vi "XYZStage Message Loop.vi"(8 "error in (no error)":errorcluster, 9 "Data Queue":refnum<queue>, 10 "Stage Readout Notifier":refnum<notifier>, 11 "Message Queues":T1) -> (0 "error out":errorcluster)   [LabVIEW 2015, in "XYZStage.lvlib"]
uses:
  XYZStage.lvlib
  support/Message Queue/All Message Queues.ctl
  support/Message Queue/Message Cluster.ctl
  XYZStage Configuration.ctl
  XYZStage State.ctl
  XYZStage Loop State.ctl
  <vilib>/Utility/error.llb/Error Cluster From Error Code.vi
  <vilib>/ErrorRing/Error Ring.xnode
  support/Message Queue/Message Queue.lvlib
panel:
  out "XYZ Microns":dbl[](array[numeric])
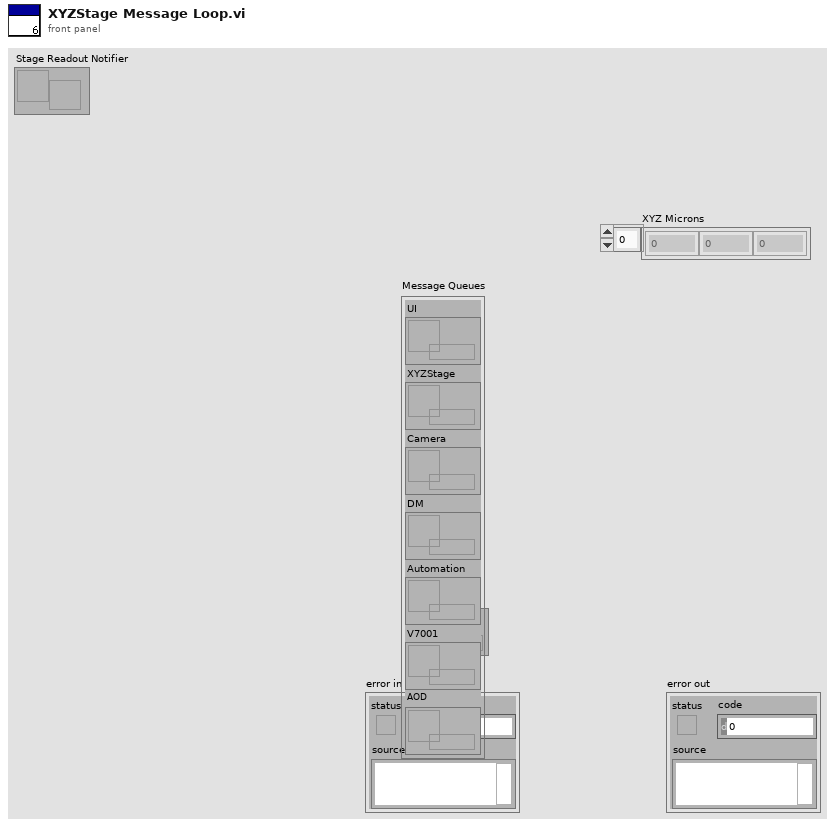
[diagram p1: front panel]
types:
  T1 = typedef "Message Queue.lvlib/All Message Queues.ctl" = cluster{"UI":refnum<queue>, "XYZStage":refnum<queue>, "Camera":refnum<queue>, "DM":refnum<queue>, "Automation":refnum<queue>, "V7001":refnum<queue>, "AOD":refnum<queue>}
  T2 = typedef "XYZStage.lvlib/XYZStage State.ctl" = cluster{"XYZStage State":T3, "Handle out":u32, "VISA resource name":refnum<visa-resource-name>, "num controllers connected":u8, "Connector statuses":u8[], "Position in Microns":dbl[], "measured manipulator":u8}
  T3 = typedef "XYZStage.lvlib/XYZStage Loop State.ctl" = enum16{"Idle", "Connected", "Moving"}
  T4 = typedef "XYZStage.lvlib/XYZStage Configuration.ctl" = cluster{"VISA resource name":refnum<visa-resource-name>, "Timeout (3sec)":u32}
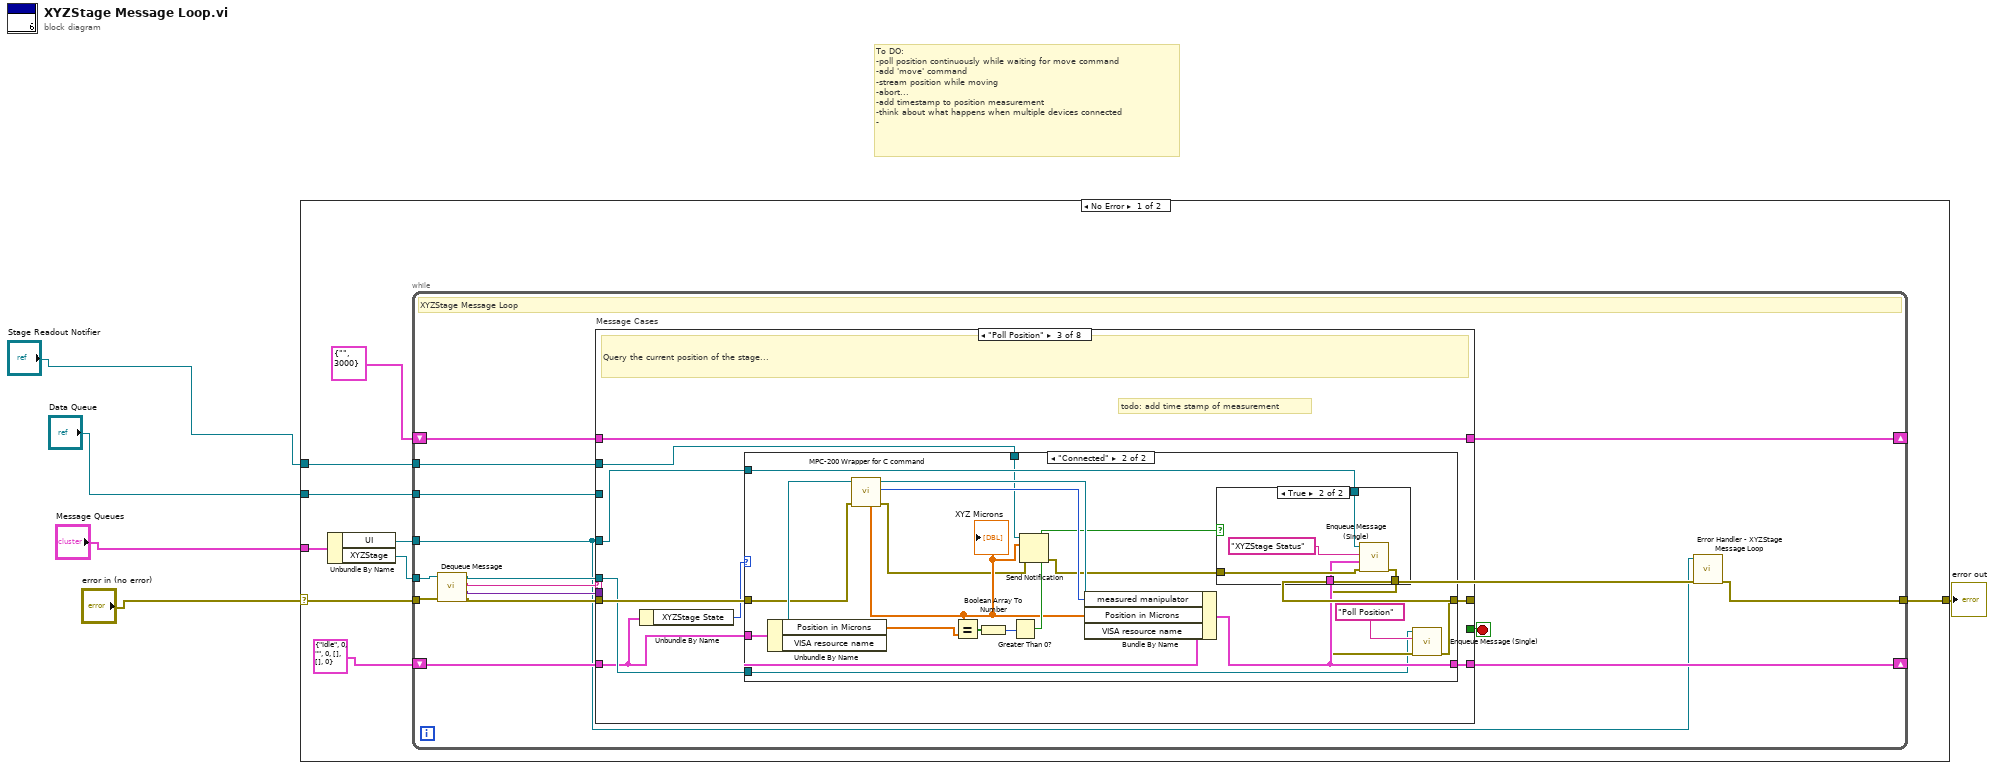
[diagram p0: block diagram]
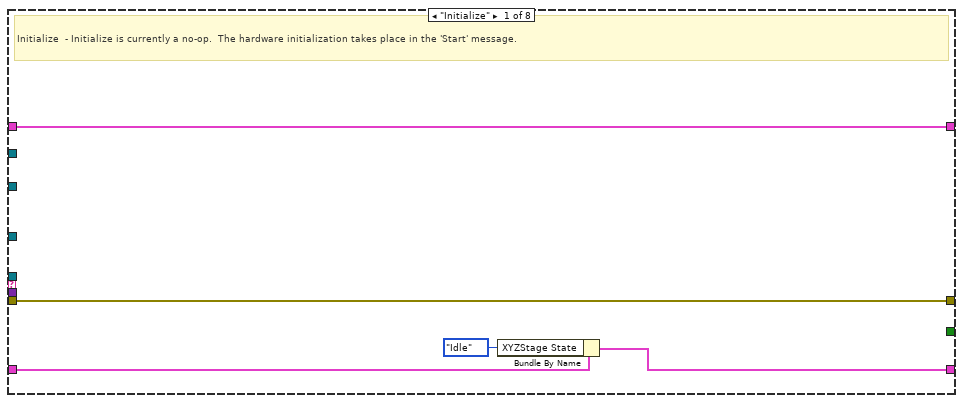
[diagram p2: hidden frame]
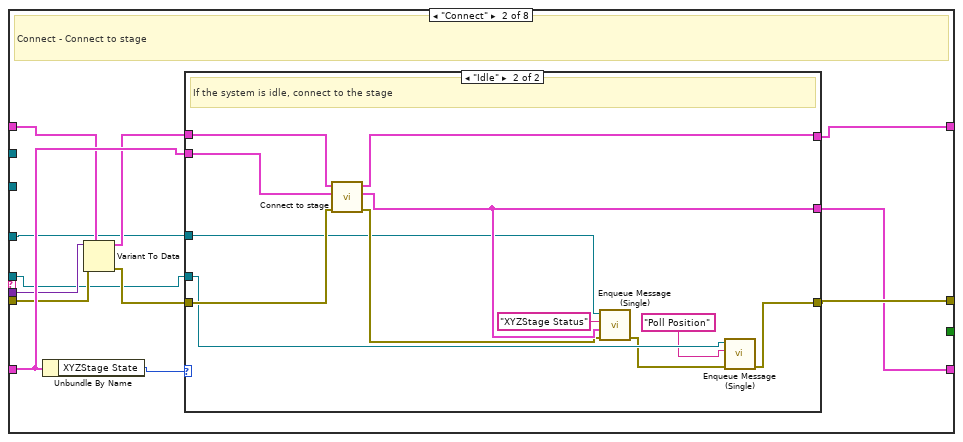
[diagram p3: hidden frame]
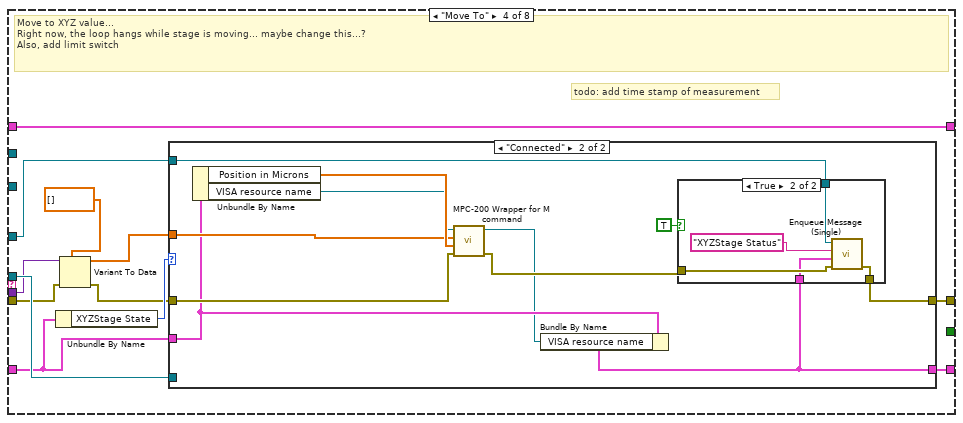
[diagram p7: hidden frame]
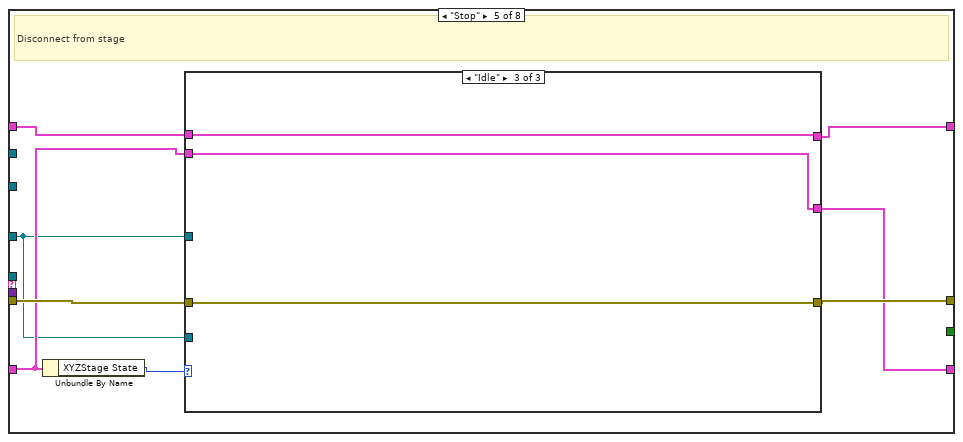
[diagram p10: hidden frame]
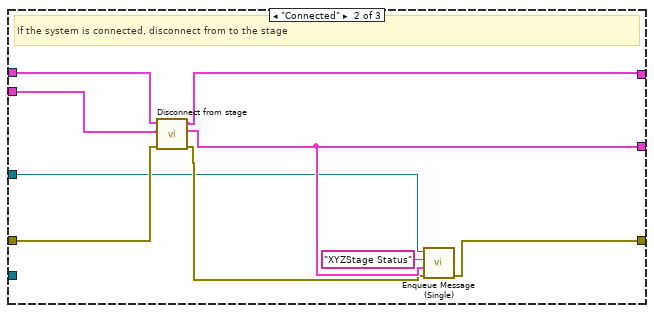
[diagram p12: hidden frame]
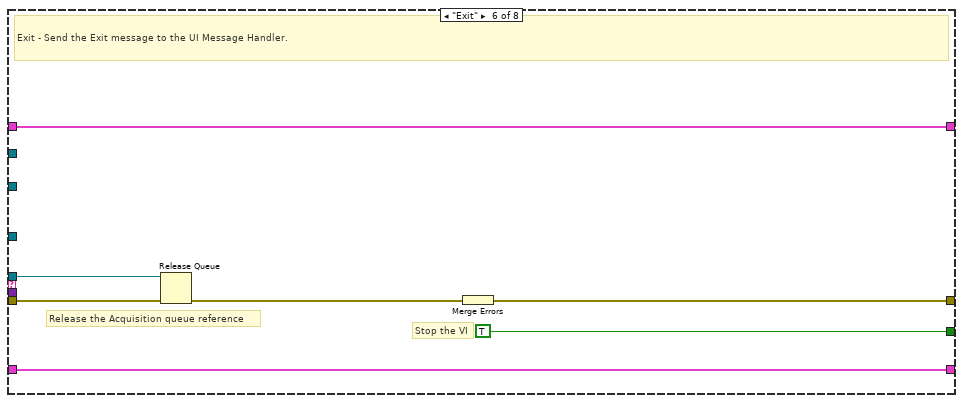
[diagram p13: hidden frame]
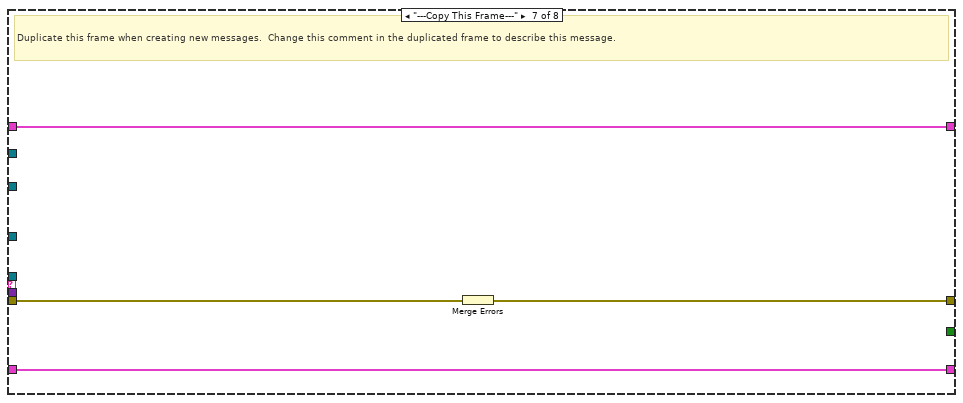
[diagram p14: hidden frame]
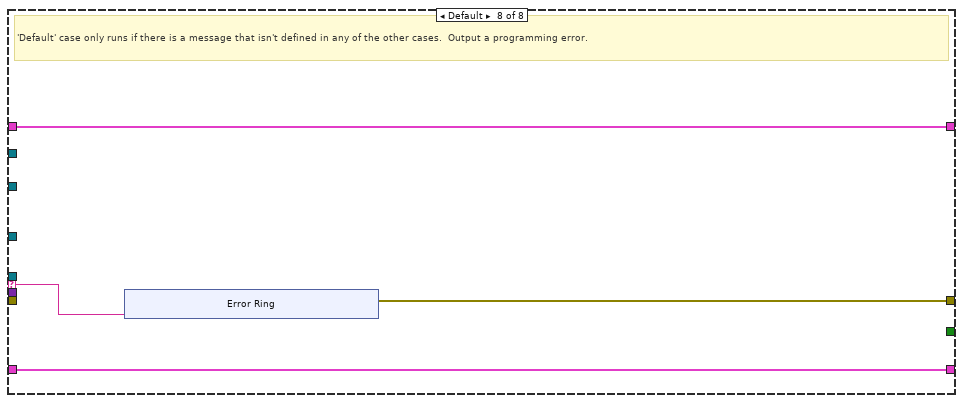
[diagram p15: hidden frame]
diagram:
  # "To DO:\n-poll position continuously while waiting for move command\n-add 'move' command\n-stream position while moving\n-abort...\n-add timestamp to position measurement\n-think about what happens when multiple devices connected\n-"
  n1 = case shown="No Error" "error in (no error)" {
    selector: "error in (no error)" -> [w11 w175]
    tunnel: "Message Queues" -> [w14 _]
    tunnel: [w12 w175] -> w5
    tunnel: "Stage Readout Notifier" -> [w9 _]
    tunnel: "Data Queue" -> [w8 _]
    frame No Error {
      n2 = Unbundle By Name(w14) -> ("UI"=w10:refnum<queue>, "XYZStage"=w13:refnum<queue>)
      n3 = while {
        tunnel: w13 -> [w23]
        shift-right: [w29] -> _
        shift-left: T4 {"VISA resource name"="", "Timeout (3sec)"=3000} ("Hardware Configuration") -> [w30]
        tunnel: w10 -> [w15]
        tunnel: w9 -> [w27]
        tunnel: w8 -> [w26]
        shift-right: [w24] -> _
        shift-left: T2 {"XYZStage State"=enum."Idle", "Handle out"=0, "VISA resource name"="", "num controllers connected"=0, "Connector statuses"=[], "Position in Microns"=[], "measured manipulator"=0} ("Cluster") -> [w25]
        tunnel: w11 -> [w22]
        tunnel: [w17] -> w12
        stop <- w28 stop-if-true
        # "XYZStage Message Loop"
        n4 = call "Dequeue Message.vi"("error in (no error)"=w22, "Message Queue"=w23) -> ("error out"=w18:errorcluster, "Message Data"=w19:variant, "Message"=w20:string, "dup Message Queue"=w21:refnum<queue>)  [unwired: 6 in]
        n5 = case "Message Cases" shown="\"Poll Position\"" w20 {
          selector: w20 -> [_ _ _ _ _ _ _ w164]
          tunnel: w21 -> [_ w36 w66 w106 _ w154 _ _]
          tunnel: w18 -> [w35 w38 w70 w103 w135 w156 w163 _]
          tunnel: [w35 w47 w67 w107 w137 w158 w161 w165] -> w16
          tunnel: w30 -> [w34 w42 w71 w110 w136 w157 w162 w167]
          tunnel: [w34 w45 w71 w110 w133 w157 w162 w167] -> w29
          tunnel: [_ _ _ _ _ TRUE _ _] -> w28
          tunnel: w19 -> [_ w40 _ w101 _ _ _ _]
          tunnel: w15 -> [_ w37 w69 w109 w130 _ _ _]
          tunnel: w27 -> [_ _ w63 _ _ _ _ _]
          tunnel: w26 -> [_ _ _ _ _ _ _ _]
          tunnel: w25 -> [w33 w43 w65 w105 w131 w153 w160 w166]
          tunnel: [w32 w46 w68 w108 w134 w153 w160 w166] -> w24
          frame "Initialize" {
            # "Initialize  - Initialize is currently a no-op.  The hardware initialization takes place in the 'Start' message."
            n6 = Bundle By Name(cluster=w33, "XYZStage State"=XYZStage_Loop_State."Idle") -> (w32:T2)
          }
          frame "Connect" {
            # "Connect - Connect to stage"
            n7 = Unbundle By Name(w43) -> ("XYZStage State"=w44:T3)
            n8 = Variant To Data(error in=w38, type=w42, Variant=w40) -> (data=w41:T4, error out=w39:errorcluster)
            n9 = case shown="\"Idle\"" w44 {
              tunnel: [w49 w51] -> w47
              tunnel: w41 -> [w50 w62]
              tunnel: w39 -> [w49 w60]
              tunnel: [w50 w61] -> w45
              tunnel: [w48 w57] -> w46
              tunnel: w43 -> [w48 w59]
              tunnel: w37 -> [_ w55]
              tunnel: w36 -> [_ w54]
              frame Default {
                # "The system is already acquiring. Ignore the \"Connect\" message."
              }
              frame "Idle" {
                # "If the system is idle, connect to the stage"
                n10 = call "Connect to stage.vi"("error in (no error)"=w60, "Hardware State"=w59, "Hardware Configuration"=w62) -> ("error out"=w56:errorcluster, "Hardware State Out"=w57:T2, "Hardware Configuration Out"=w61:T4)  [unwired: 6 in]
                n11 = call "Enqueue Message (Single).vi"("error in (no error)"=w56, "Message Data"=w57, "Message"="XYZStage Status", "Message Queue"=w55) -> ("error out"=w52:errorcluster)  [unwired: 6 in, 1 out]
                n12 = call "Enqueue Message (Single).vi"("error in (no error)"=w52, "Message"="Poll Position", "Message Queue"=w54) -> ("error out"=w51:errorcluster)  [unwired: 7 in, 1 out]
              }
            }
          }
          frame "Poll Position" {
            # "todo: add time stamp of measurement"
            # "Query the current position of the stage..."
            n13 = Unbundle By Name(w65) -> ("XYZStage State"=w64:T3)
            n14 = case shown="\"Connected\"" w64 {
              tunnel: w70 -> [w73 w91]
              tunnel: w65 -> [w72 w90]
              tunnel: w69 -> [_ w87]
              tunnel: [w72 w86] -> w68
              tunnel: [w73 w81] -> w67
              tunnel: w66 -> [_ w78]
              tunnel: w63 -> [_ w77]
              frame "Idle", Default {
              }
              frame "Connected" {
                n15 = Unbundle By Name(w90) -> ("Position in Microns"=w85:dbl[], "VISA resource name"=w92:refnum<visa-resource-name>)
                n16 = call "MPC-200 Wrapper for C command.vi"("error in (no error)"=w91, "VISA resource name in"=w92) -> ("error out"=w75:errorcluster, "Manipulator Number"=w88:u8, "VISA resource name out"=w89:refnum<visa-resource-name>, "XYZ Microns"=w76:dbl[])  [unwired: 5 in, 1 out]
                "XYZ Microns" <- w76
                n17 = Equal?(x=w76, y=w85) -> (x = y?=w84:bool[])
                n18 = Boolean Array To Number(Boolean array=w84) -> (number=w83:u32)
                n19 = Greater Than 0?(x=w83) -> (x > 0?=w82:bool)
                n20 = Send Notification(notification=w76, notifier=w77, error in (no error)=w75) -> (error out=w74:errorcluster)  [unwired: 1 out]
                n21 = Bundle By Name(cluster=w90, "measured manipulator"=w88, "Position in Microns"=w76, "VISA resource name"=w89) -> (w86:T2)
                n22 = case shown="True" w82 {
                  tunnel: w87 -> [_ w97]
                  tunnel: w74 -> [w93 w96]
                  tunnel: [w93 w95] -> w80
                  tunnel: w86 -> [_ w94]
                  frame False {
                  }
                  frame True {
                    n23 = call "Enqueue Message (Single).vi"("error in (no error)"=w96, "Message Data"=w94, "Message"="XYZStage Status", "Message Queue"=w97) -> ("error out"=w95:errorcluster)  [unwired: 6 in, 1 out]
                  }
                }
                n24 = call "Enqueue Message (Single).vi"("error in (no error)"=w80, "Message"="Poll Position", "Message Queue"=w78) -> ("error out"=w81:errorcluster)  [unwired: 7 in, 1 out]
              }
            }
          }
          frame "Move To" {
            # "todo: add time stamp of measurement"
            # "Move to XYZ value...\nRight now, the loop hangs while stage is moving... maybe change this...?\nAlso, add limit switch"
            n25 = Unbundle By Name(w105) -> ("XYZStage State"=w104:T3)
            n26 = Variant To Data(error in=w103, type=dbl[] [] ("XYZ Microns"), Variant=w101) -> (data=w99:dbl[], error out=w102:errorcluster)
            n27 = case shown="\"Connected\"" w104 {
              tunnel: w102 -> [w112 w119]
              tunnel: w105 -> [w111 w117]
              tunnel: w109 -> [_ w123]
              tunnel: [w111 w116] -> w108
              tunnel: [w112 w114] -> w107
              tunnel: w106 -> [_ _]
              tunnel: w99 -> [_ w120]
              frame "Idle", Default {
              }
              frame "Connected" {
                n28 = Unbundle By Name(w117) -> ("Position in Microns"=w122:dbl[], "VISA resource name"=w121:refnum<visa-resource-name>)
                n29 = call "MPC-200 Wrapper for M command.vi"("error in (no error)"=w119, "Current Position"=w122, "Move to Position"=w120, "VISA resource name in"=w121) -> ("error out"=w118:errorcluster, "VISA resource name out"=w115:refnum<visa-resource-name>)  [unwired: 6 in]
                n30 = Bundle By Name(cluster=w117, "VISA resource name"=w115) -> (w116:T2)
                n31 = case shown="True" TRUE {
                  tunnel: w123 -> [_ w128]
                  tunnel: w118 -> [w124 w127]
                  tunnel: [w124 w126] -> w114
                  tunnel: w116 -> [_ w125]
                  frame False {
                  }
                  frame True {
                    n32 = call "Enqueue Message (Single).vi"("error in (no error)"=w127, "Message Data"=w125, "Message"="XYZStage Status", "Message Queue"=w128) -> ("error out"=w126:errorcluster)  [unwired: 6 in, 1 out]
                  }
                }
              }
            }
          }
          frame "Stop" {
            # "Disconnect from stage"
            n33 = Unbundle By Name(w131) -> ("XYZStage State"=w132:T3)
            n34 = case shown="\"Idle\"" w132 {
              tunnel: [w139 w148 w152] -> w137
              tunnel: w136 -> [w140 w142 w151]
              tunnel: w135 -> [w139 w144 w152]
              tunnel: [w140 w147 w151] -> w133
              tunnel: [w138 w146 w150] -> w134
              tunnel: w130 -> [_ _ _]
              tunnel: w131 -> [w138 w143 w150]
              tunnel: w130 -> [_ w141 _]
              frame Default {
                # "The system is already acquiring. Ignore the \"Connect\" message."
              }
              frame "Connected" {
                # "If the system is connected, disconnect from to the stage"
                n35 = call "Disconnect from stage.vi"("error in (no error)"=w144, "Hardware State"=w143, "Hardware Configuration"=w142) -> ("error out"=w145:errorcluster, "Hardware State Out"=w146:T2, "Hardware Configuration Out"=w147:T4)  [unwired: 6 in]
                n36 = call "Enqueue Message (Single).vi"("error in (no error)"=w145, "Message Data"=w146, "Message"="XYZStage Status", "Message Queue"=w141) -> ("error out"=w148:errorcluster)  [unwired: 6 in, 1 out]
              }
              frame "Idle" {
              }
            }
          }
          frame "Exit" {
            # "Release the Acquisition queue reference"
            # "Stop the VI"
            # "Exit - Send the Exit message to the UI Message Handler."
            n37 = Release Queue(queue=w154, error in (no error)=w156) -> (error out=w155:errorcluster)  [unwired: 1 in, 2 out]
            n38 = Merge Errors(w155) -> (w158:errorcluster)
          }
          frame "---Copy This Frame---" {
            # "Duplicate this frame when creating new messages.  Change this comment in the duplicated frame to describe this message."
            n39 = Merge Errors(w163) -> (w161:errorcluster)
          }
          frame Default {
            # "'Default' case only runs if there is a message that isn't defined in any of the other cases.  Output a programming error."
            n40 = xnode "Error Ring"("parameter 0"=w164) -> ("error out"=w165:errorcluster)
          }
        }
        n41 = call "Error Handler - XYZStage Message Loop.vi"("error in (no error)"=w16, "Message Queue"=w15) -> ("dup error in"=w17:errorcluster)  [unwired: 8 in, 1 out]
      }
    }
    frame Error {
    }
  }
  "error out" <- w5
